vi "Write initial setup.vi"(8 "error in (no error)":errorcluster, 11 "Channel in":refnum<class "Channel.lvclass">) -> (0 "error out":errorcluster, 3 "Channel out":refnum<class "Channel.lvclass">)   [LabVIEW 2018, in "Channel.lvclass"]
uses:
  Channel.lvclass
  Channel.lvclass/Channel.ctl
  <vilib>/Utility/config.llb/Write Key (Boolean).vi
  <vilib>/Utility/config.llb/Write Key (String).vi
  <vilib>/Utility/config.llb/NI_LVConfig.lvlib
panel:
  out "ACS configuration":T1
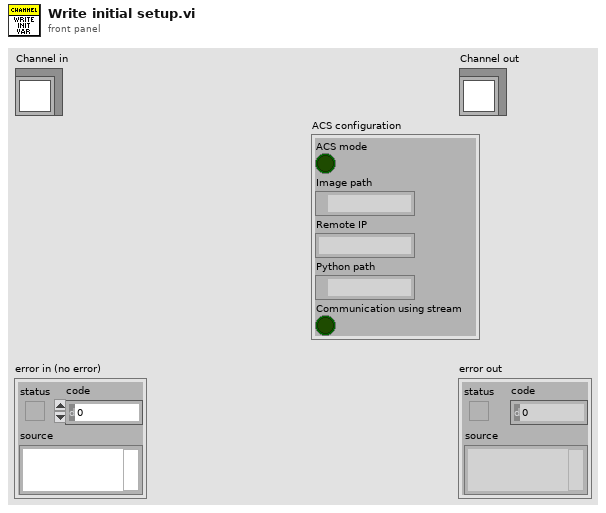
[diagram p1: front panel]
types:
  T1 = cluster{"ACS mode":bool, "Image path":path, "Remote IP":string, "Python path":path, "Communication using stream":bool}
  T2 = typedef "NI_LVConfig.lvlib/Config Data RefNum.ctl" = refnum<k1>
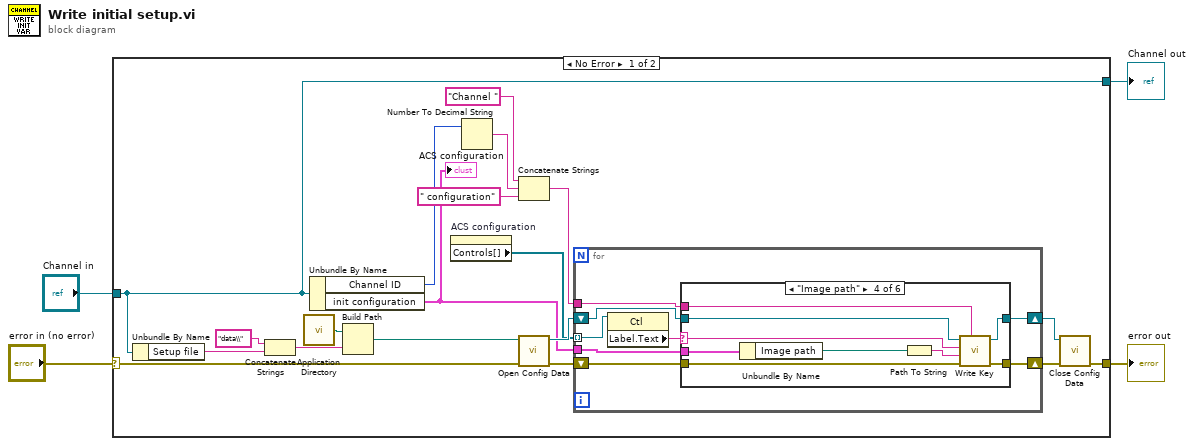
[diagram p0: block diagram]
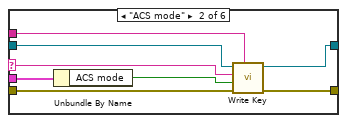
[diagram p3: hidden frame]
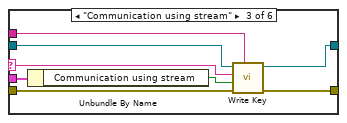
[diagram p4: hidden frame]
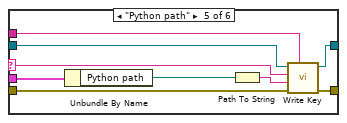
[diagram p5: hidden frame]
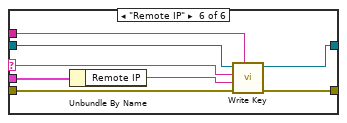
[diagram p6: hidden frame]
diagram:
  n1 = case shown="No Error" "error in (no error)" {
    selector: "error in (no error)" -> [w21 w77]
    tunnel: [w20 w77] -> w3
    tunnel: [w12 w76] -> w1
    tunnel: "Channel in" -> [w12 w76]
    frame No Error {
      n2 = Unbundle By Name(w12) -> ("Setup file"=w10:string)
      n3 = Concatenate Strings("data\\", w10) -> (w11:string)
      n4 = call <vilib>:"Application Directory.vi"() -> ("Application Directory"=w23:path)
      n5 = Unbundle By Name(w12) -> ("Channel ID"=w16:u8, "init configuration"=w6:T1)
      "ACS configuration" <- w6
      n6 = Build Path(base path=w23, name or relative path=w11) -> (appended path=w22:path)
      n7 = property on="ACS configuration" class="Clust (strict)"() -> ("Controls[]"=w5:refnum<vi>[])  [unwired: 2 in, 2 out]
      n8 = Number To Decimal String(number=w16) -> (decimal integer string=w14:string)  [unwired: 1 in]
      n9 = Concatenate Strings("Channel ", w14, " configuration") -> (w13:string)
      n10 = call <vilib>:"Open Config Data.vi"("error in (no error)"=w21, "configuration file path"=w22) -> ("error out"=w8:errorcluster, "refnum"=w17:T2)  [unwired: 7 in, 1 out]
      n11 = for {
        tunnel: w13 -> [w28]
        shift-right: [w30] -> w18
        shift-left: w17 -> [w29]
        shift-right: [w31] -> w19
        shift-left: w8 -> [w27]
        tunnel: w6 -> [w26]
        tunnel: w5 -> [w25] mode=indexing
        n12 = property class="Ctl"(reference=w25) -> ("Label.Text"=w24:string)  [unwired: 1 in, 2 out]
        n13 = case shown="\"Image path\"" w24 {
          selector: w24 -> [_ w35 w42 w51 w60 w69]
          tunnel: [w32 w41 w49 w58 w67 w75] -> w31
          tunnel: [w33 w40 w48 w57 w66 w74] -> w30
          tunnel: w29 -> [w33 w39 w47 w56 w65 w73]
          tunnel: w28 -> [_ w38 w46 w55 w64 w72]
          tunnel: w27 -> [w32 w37 w45 w54 w63 w71]
          tunnel: w26 -> [_ w34 w43 w50 w59 w68]
          frame "False", Default {
          }
          frame "ACS mode" {
            n14 = Unbundle By Name(w34) -> ("ACS mode"=w36:bool)
            n15 = call-poly <vilib>:"Write Key.vi"("section"=w38, "error in (no error)"=w37, "value"=w36, "key"=w35, "refnum"=w39) -> ("error out"=w41:errorcluster, "refnum out"=w40:T2)  [unwired: 4 in, 1 out]
          }
          frame "Communication using stream" {
            n16 = Unbundle By Name(w43) -> ("Communication using stream"=w44:bool)
            n17 = call-poly <vilib>:"Write Key.vi"("section"=w46, "error in (no error)"=w45, "value"=w44, "key"=w42, "refnum"=w47) -> ("error out"=w49:errorcluster, "refnum out"=w48:T2)  [unwired: 4 in, 1 out]
          }
          frame "Image path" {
            n18 = Unbundle By Name(w50) -> ("Image path"=w53:path)
            n19 = Path To String(path=w53) -> (string=w52:string)
            n20 = call-poly <vilib>:"Write Key.vi"("section"=w55, "error in (no error)"=w54, "value"=w52, "key"=w51, "refnum"=w56) -> ("error out"=w58:errorcluster, "refnum out"=w57:T2)  [unwired: 4 in, 1 out]
          }
          frame "Python path" {
            n21 = Unbundle By Name(w59) -> ("Python path"=w62:path)
            n22 = Path To String(path=w62) -> (string=w61:string)
            n23 = call-poly <vilib>:"Write Key.vi"("section"=w64, "error in (no error)"=w63, "value"=w61, "key"=w60, "refnum"=w65) -> ("error out"=w67:errorcluster, "refnum out"=w66:T2)  [unwired: 4 in, 1 out]
          }
          frame "Remote IP" {
            n24 = Unbundle By Name(w68) -> ("Remote IP"=w70:string)
            n25 = call-poly <vilib>:"Write Key.vi"("section"=w72, "error in (no error)"=w71, "value"=w70, "key"=w69, "refnum"=w73) -> ("error out"=w75:errorcluster, "refnum out"=w74:T2)  [unwired: 4 in, 1 out]
          }
        }
      }
      n26 = call <vilib>:"Close Config Data.vi"("error in (no error)"=w19, "refnum"=w18) -> ("error out"=w20:errorcluster)  [unwired: 8 in, 1 out]
    }
    frame Error {
    }
  }
  "error out" <- w3
  "Channel out" <- w1
